vi "Buffer printing.vi"(8 "error in (no error)":errorcluster, 11 "Domino Laser module Class in":refnum<class "Domino Laser module Class.lvclass">) -> (0 "error out":errorcluster, 3 "Domino Laser module Class out":refnum<class "Domino Laser module Class.lvclass">)   [LabVIEW 2024, in "Domino LM.lvlib" / "Domino Laser module Class.lvclass"]
uses:
  CTRLS/Domino Laser module Class.lvclass
  ARCH/Message Queue/Message Cluster.ctl
  CTRLS/Domino Laser module Class.lvclass/Domino Laser module Class.ctl
  <vilib>/Utility/error.llb/Trim Whitespace One-Sided.vi
  CTRLS/GLB_VAR.vi
  ARCH/Message Queue/Message Queue.lvlib
panel:
  out "Printer Serial Array":string[](array[string])
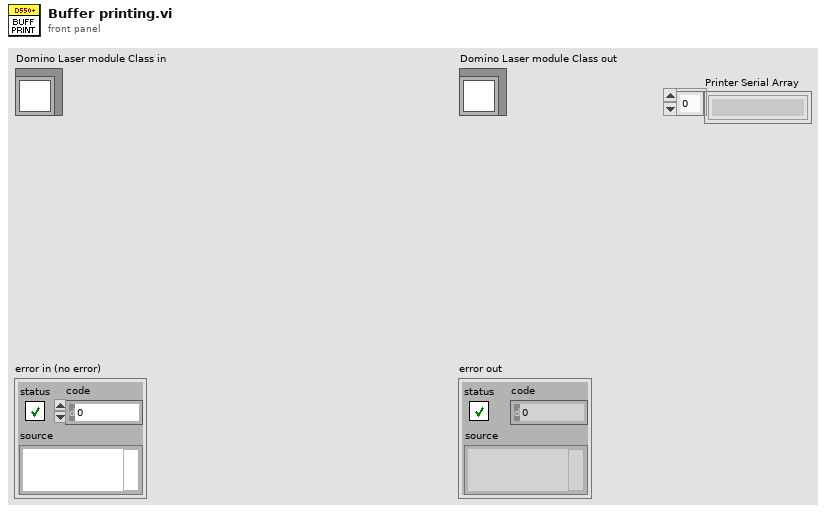
[diagram p1: front panel]
types:
  T1 = enum16{"Send variable to print", "Wait for print end", "INIT", "Send 2 first serials"}
  T2 = typedef "Message Queue.lvlib/Message Cluster.ctl" = cluster{"Message":string, "Message Data":variant}
  T3 = enum16{"Send variable to print", "Wait for print end", "INIT"}
  T4 = enum16{"Init SRL Buffer", "Insert SRL in Buffer", "Insert SRL Status", "Remove SRL from Buffer"}
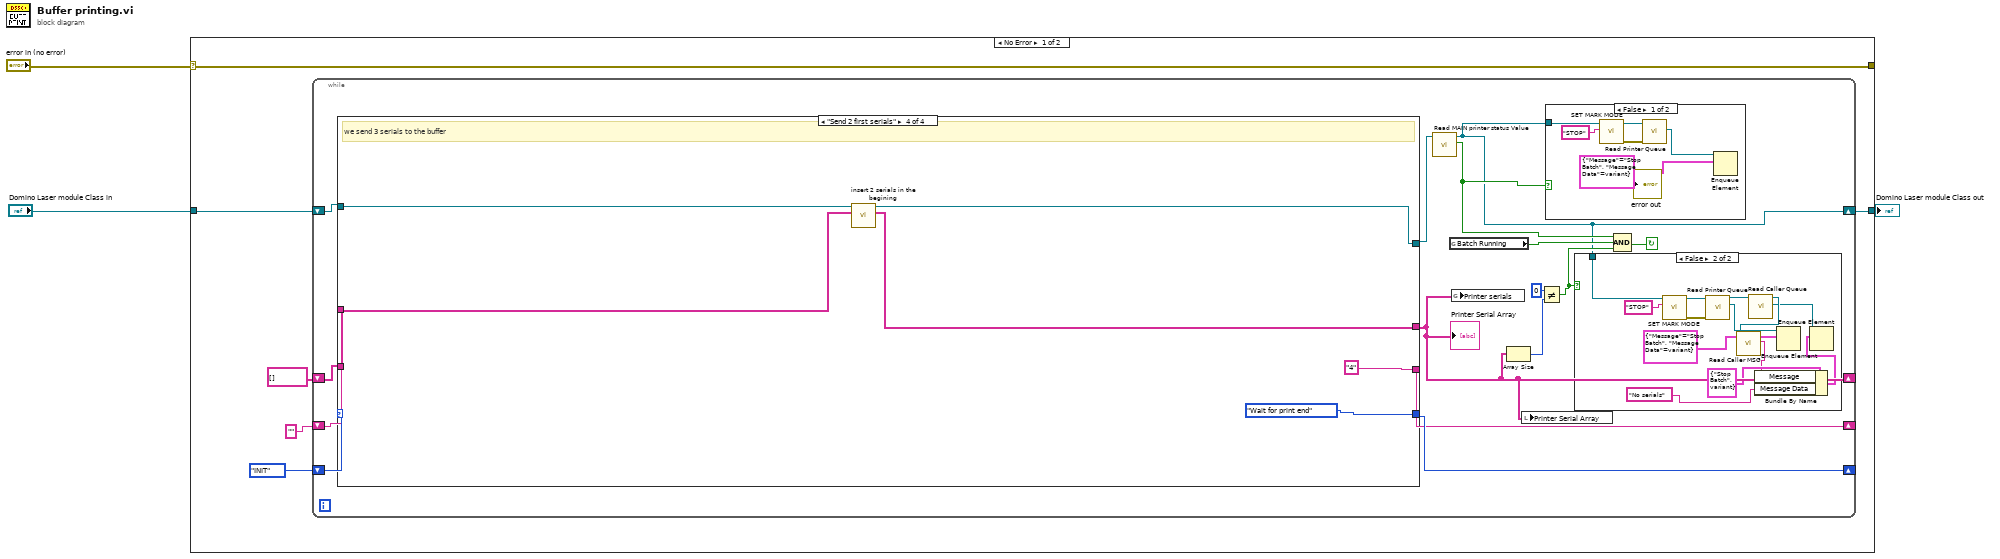
[diagram p0: block diagram]
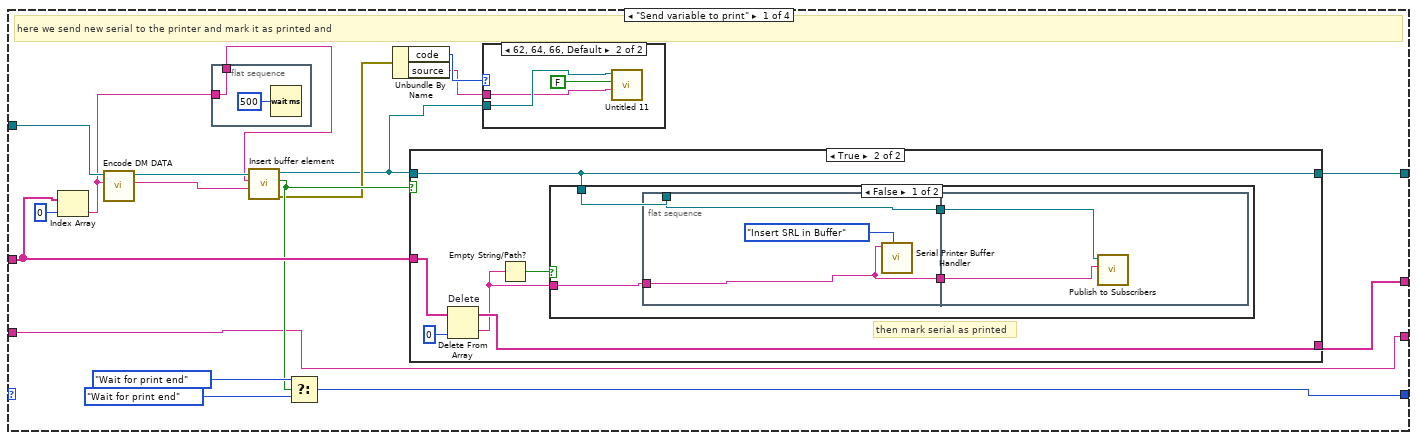
[diagram p4: hidden frame]
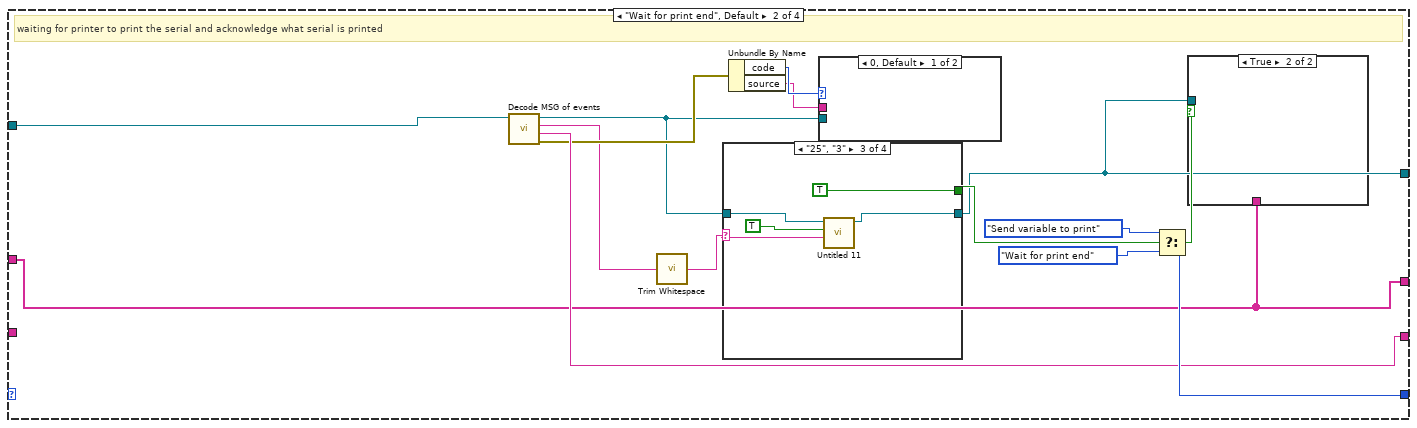
[diagram p8: hidden frame]
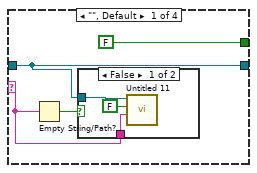
[diagram p10: hidden frame]
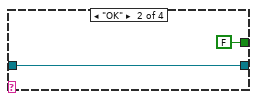
[diagram p12: hidden frame]
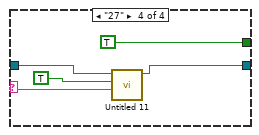
[diagram p13: hidden frame]
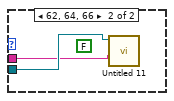
[diagram p14: hidden frame]
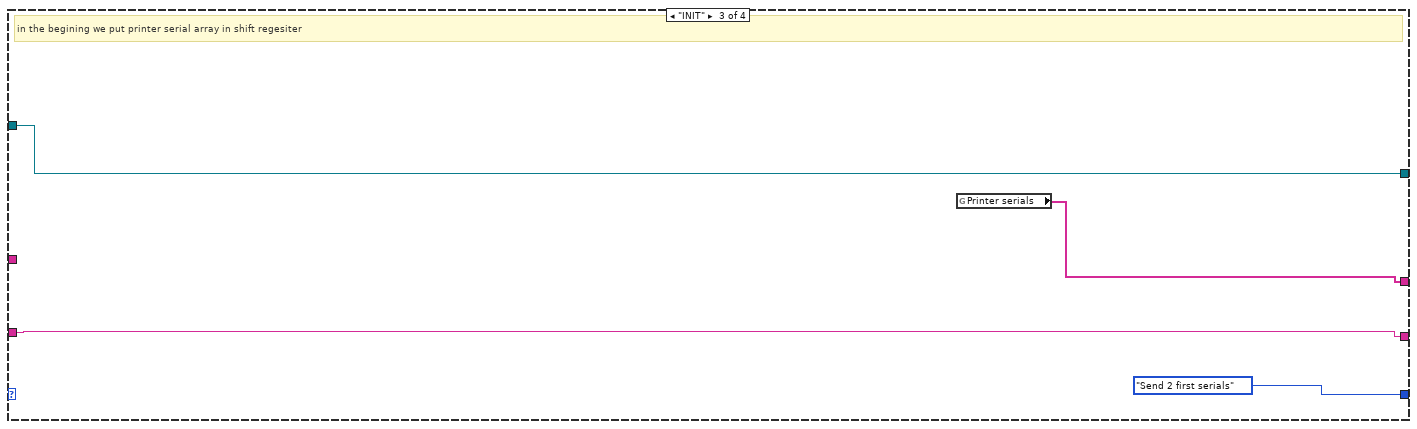
[diagram p15: hidden frame]
diagram:
  n1 = case shown="No Error" "error in (no error)" {
    selector: "error in (no error)" -> [w9 w130]
    tunnel: [w9 w130] -> _
    tunnel: [w8 w129] -> w2
    tunnel: "Domino Laser module Class in" -> [w6 w129]
    frame No Error {
      n2 = while {
        shift-right: [w10] -> w8
        shift-left: w6 -> [w24]
        shift-right: [w13] -> _
        shift-left: string[] [] ("Seials array") -> [w23]
        shift-right: [w20] -> _
        shift-left: T1."INIT" ("Enum") -> [w21]
        shift-right: [w16] -> _
        shift-left: "" -> [w17]
        stop <- w18 continue-if-true
        n3 = case shown="\"Send 2 first serials\"" w21 {
          tunnel: w24 -> [w54 w97 w122 w128]
          tunnel: [w60 w85 w122 w127] -> w22
          tunnel: w23 -> [w59 w84 _ w124]
          tunnel: [w55 w84 w119 w123] -> w13
          tunnel: [w56 w94 T1."Send 2 first serials" ("Enum") T3."Wait for print end" ("Enum")] -> w20
          tunnel: w17 -> [w50 _ w120 _]
          tunnel: [w50 w93 w120 "4" ("buffer ID")] -> w16
          frame "Send variable to print" {
            # "here we send new serial to the printer and mark it as printed and"
            n4 = Index Array(array=w59, index=0) -> (element=w45:string)
            n5 = call "Encode DM DATA.vi"("serial"=w45, "Domino Laser module Class in"=w54) -> ("DM"=w52:string, "Domino Laser module Class out"=w53:refnum<class "Domino Laser module Class.lvclass">)  [unwired: 7 in, 1 out]
            n6 = flat-sequence {
              tunnel: w45 -> [w62]
              tunnel: [w62] -> w44
              frame #0 {
                n7 = Wait (ms)(milliseconds to wait=u32 500) -> ()  [unwired: 1 out]
              }
            }
            n8 = call "Insert buffer element.vi"("DM"=w52, "Serial"=w44, "Domino Laser module Class in"=w53) -> ("error out"=w47:errorcluster, "element inserted successfully"=w51:bool, "Domino Laser module Class out"=w46:refnum<class "Domino Laser module Class.lvclass">)  [unwired: 6 in]
            n9 = Select(t=T3."Wait for print end" ("Enum"), s=w51, f=T3."Wait for print end" ("Enum")) -> (s? t:f=w56:T3)
            n10 = Unbundle By Name(w47) -> ("code"=w49:i32, "source"=w48:string)
            n11 = case shown="True" w51 {
              tunnel: [w68 w69] -> w60
              tunnel: w46 -> [w68 w69]
              tunnel: w59 -> [w67 w73]
              tunnel: [w67 w72] -> w55
              frame False {
              }
              frame True {
                # "then mark serial as printed"
                n12 = Delete From Array "Delete"(array=w73, index=0) -> (deleted portion=w70:string, array with subset deleted=w72:string[])  [unwired: 1 in]
                n13 = Empty String/Path?(string/path=w70) -> (empty?=w71:bool)
                n14 = case shown="False" w71 {
                  tunnel: w70 -> [w78 _]
                  tunnel: w69 -> [w77 _]
                  frame False {
                    n15 = flat-sequence {
                      tunnel: w78 -> [w79]
                      tunnel: w77 -> [w81]
                      tunnel: [w81] -> w76
                      tunnel: [w79] -> w75
                      tunnel: w76 -> [w83]
                      tunnel: w75 -> [w82]
                      frame #0 {
                        n16 = call "Serial Printer Buffer Handler.vi"("Serials buffer operations"=T4."Insert SRL in Buffer", "Serial"=w79) -> ()  [unwired: 8 in, 2 out]
                      }
                      frame #1 {
                        n17 = call "Publish to Subscribers.vi"("Message Data"=w82, "Domino Laser module Class in"=w83) -> ()  [unwired: 8 in, 2 out]
                      }
                    }
                  }
                  frame True {
                  }
                }
              }
            }
            n18 = case shown="62, 64, 66, Default" w49 {
              tunnel: w46 -> [_ w66]
              tunnel: w48 -> [_ w64]
              frame 0 {
              }
              frame 62, 64, 66, Default {
                n19 = call "Untitled 11.vi"("MSG"=w64, "MSG Status"=FALSE, "Domino Laser module Class in"=w66) -> ()  [unwired: 7 in, 2 out]
              }
            }
          }
          frame "Wait for print end", Default {
            # "waiting for printer to print the serial and acknowledge what serial is printed"
            n20 = call "Decode MSG of events.vi"("Domino Laser module Class in"=w97) -> ("error out"=w90:errorcluster, "buffer ID"=w93:string, "MSG ID"=w88:string, "Domino Laser module Class out"=w89:refnum<class "Domino Laser module Class.lvclass">)  [unwired: 7 in]
            n21 = call <vilib>:"Trim Whitespace.vi"("string"=w88) -> ("trimmed string"=w87:string)  [unwired: 1 in]
            n22 = case shown="\"25\", \"3\"" w87 {
              selector: w87 -> [w98 _ w107 w112]
              tunnel: [FALSE FALSE TRUE TRUE] -> w86
              tunnel: w89 -> [w100 w105 w110 w115]
              tunnel: [w100 w105 w109 w114] -> w85
              frame "", Default {
                n23 = Empty String/Path?(string/path=w98) -> (empty?=w99:bool)
                n24 = case shown="False" w99 {
                  tunnel: w100 -> [w104 _]
                  tunnel: w98 -> [w102 _]
                  frame False {
                    n25 = call "Untitled 11.vi"("MSG"=w102, "MSG Status"=FALSE, "Domino Laser module Class in"=w104) -> ()  [unwired: 7 in, 2 out]
                  }
                  frame True {
                  }
                }
              }
              frame "OK" {
              }
              frame "25", "3" {
                n26 = call "Untitled 11.vi"("MSG"=w107, "MSG Status"=TRUE, "Domino Laser module Class in"=w110) -> ("Domino Laser module Class out"=w109:refnum<class "Domino Laser module Class.lvclass">)  [unwired: 7 in, 1 out]
              }
              frame "27" {
                n27 = call "Untitled 11.vi"("MSG"=w112, "MSG Status"=TRUE, "Domino Laser module Class in"=w115) -> ("Domino Laser module Class out"=w114:refnum<class "Domino Laser module Class.lvclass">)  [unwired: 7 in, 1 out]
              }
            }
            n28 = Unbundle By Name(w90) -> ("code"=w92:i32, "source"=w91:string)
            n29 = case shown="0, Default" w92 {
              tunnel: w89 -> [_ w118]
              tunnel: w91 -> [_ w117]
              frame 0, Default {
              }
              frame 62, 64, 66 {
                (unwired) FALSE ("MSG Status")
                n30 = call "Untitled 11.vi"("MSG"=w117, "Domino Laser module Class in"=w118) -> ()  [unwired: 8 in, 2 out]
              }
            }
            n31 = Select(t=T3."Send variable to print" ("Enum"), s=w86, f=T3."Wait for print end" ("Enum")) -> (s? t:f=w94:T3)
            n32 = case shown="True" w86 {
              tunnel: w85 -> [_ _]
              tunnel: w84 -> [_ _]
              frame False {
              }
              frame True {
              }
            }
          }
          frame "INIT" {
            # "in the begining we put printer serial array in shift regesiter"
            n33 = global read "GLB_VAR.vi" "Printer serials"() -> (w119:string[])
          }
          frame "Send 2 first serials" {
            # "we send 3 serials to the buffer"
            n34 = call "insert 2 serials in the begining.vi"("Seials array"=w124, "Domino Laser module Class in"=w128) -> ("array w/ subset deleted"=w123:string[], "Domino Laser module Class out"=w127:refnum<class "Domino Laser module Class.lvclass">)  [unwired: 7 in, 1 out]
          }
        }
        "Printer Serial Array" <- w13
        n35 = call "Read MAIN printer status Value.vi"("Domino Laser module Class in"=w22) -> ("Print stat"=w12:bool, "Domino Laser module Class out"=w10:refnum<class "Domino Laser module Class.lvclass">)  [unwired: 8 in, 1 out]
        n36 = global read "GLB_VAR.vi" "Batch Running"() -> (w19:bool)
        n37 = global write "GLB_VAR.vi" "Printer serials"(w13) -> ()
        n38 = Array Size(array=w13) -> (size(s)=w15:i32)
        n39 = local write "Printer Serial Array"(w13) -> ()
        n40 = Not Equal?(x=0, y=w15) -> (x != y?=w11:bool)
        n41 = case shown="False" w12 {
          tunnel: w10 -> [w43 _]
          frame False {
            n42 = call "SET MARK MODE.vi"("mark mode"="STOP", "Domino Laser module Class in"=w43) -> ("error out"=w41:errorcluster, "Domino Laser module Class out"=w40:refnum<class "Domino Laser module Class.lvclass">)  [unwired: 8 in]
            n43 = call "Read Printer Queue.vi"("error in (no error)"=w41, "Domino Laser module Class in"=w40) -> ("Printer Queue"=w39:refnum<queue>)  [unwired: 7 in, 2 out]
            n44 = Enqueue Element(queue=w39, element=T2 {"Message"="Stop Batch", "Message Data"=variant}) -> ()  [unwired: 2 in, 3 out]
          }
          frame True {
          }
        }
        n45 = case shown="False" w11 {
          tunnel: w10 -> [_ w32]
          frame True {
          }
          frame False {
            n46 = call "SET MARK MODE.vi"("mark mode"="STOP", "Domino Laser module Class in"=w32) -> ("error out"=w36:errorcluster, "Domino Laser module Class out"=w35:refnum<class "Domino Laser module Class.lvclass">)  [unwired: 8 in]
            n47 = call "Read Printer Queue.vi"("error in (no error)"=w36, "Domino Laser module Class in"=w35) -> ("Printer Queue"=w34:refnum<queue>, "Domino Laser module Class out"=w31:refnum<class "Domino Laser module Class.lvclass">)  [unwired: 7 in, 1 out]
            n48 = call "Read Caller Queue.vi"("Domino Laser module Class in"=w31) -> ("Caller Queue"=w29:refnum<queue>, "Domino Laser module Class out"=w30:refnum<class "Domino Laser module Class.lvclass">)  [unwired: 8 in, 1 out]
            n49 = call "Read Caller MSG.vi"("Domino Laser module Class in"=w30) -> ("Caller MSG"=w27:string)  [unwired: 8 in, 2 out]
            n50 = Bundle By Name(cluster=T2 {"Message"="Stop Batch", "Message Data"=variant} ("element"), "Message"=w27, "Message Data"="No serials" ("mark mode")) -> (w25:T2)
            n51 = Enqueue Element(queue=w34, element=T2 {"Message"="Stop Batch", "Message Data"=variant}) -> ()  [unwired: 2 in, 3 out]
            n52 = Enqueue Element(queue=w29, element=w25) -> ()  [unwired: 2 in, 3 out]
          }
        }
        n53 = Compound Arithmetic op=AND(w12, w19, w11) -> (w18:bool)
      }
    }
    frame Error {
    }
  }
  "Domino Laser module Class out" <- w2
